vi "RX Detect Sync Error.vi"(0 "rx baseband session in":T2={"3630 session"={"VISA resource name"="", "Address Space"=1, "window_offset"=0, "register_addresses"={"MM based Registers"={"Revision"=0, "OldestCompatRev"=0, "signature"=0, "scratch"=0, "LedControl"=0, "BoardHwRev"=0, "BoardControl"=0, "ThermalStatus"=0, "BasebandStatus"=0, "BasebandControl"=0, "BasebandAuxSetup"=0, "BasebandAuxStatus"=0, "LmkSyncOutSetup"=0, " AdcSyncOutSetup"=0, " InjSyncOutSetup"=0, " PxiTrig0OutSetup"=0, " PxiTrig1OutSetup"=0, " PxiTrig2OutSetup"=0, " PxiTrig3OutSetup"=0, " PxiTrig4OutSetup"=0, " PxiTrig5OutSetup"=0, " PxiTrig6OutSetup"=0, " PxiTrig7OutSetup"=0}, "CPLD based Registers"={"SlaveSignature"=0, "SlaveRevision"=0, "SlaveOldestCompatRev"=0, "SlaveScratch"=0, "SlaveSetup"=0, "SlaveStatus"=0, "IDacReg_offset"=0, "LMKRegGrp0_offset"=0, "QDacReg_offset"=0, "BrdTempSensorVal"=0, "TempSensorPowerDown"=0, "GPIOReg_offset"=0, "IAdcReg_offset"=0, "QAdcReg_offset"=0, "LMKRegGrp1_offset"=0, "QadcTempSensorVal"=0, "IadcTempSensorVal"=0, "RevisionReg"=0, "VcxoReg"=0, "CpldStatusReg"=0, "PowerReg"=0, "VBiasEnReg"=0, "ExtRefOeReg"=0, "QdacCtrlReg"=0, "QdacStatusReg"=0, "IdacCtrlReg"=0, "IdacStatusReg"=0, "QdacJtagIn"=0, "QdacJtagOut"=0, "IdacJtagIn"=0, "IdacJtagOut"=0, "IqDcSetupReg"=0, "QadcStatusReg"=0, "IadcStatusReg"=0, "BrdSetupReg"=0, "IqDcRevisionReg"=0, "PllStatusReg"=0, "EndpointScratchReg"=0, "AdcSyncCfgReg"=0, "IqCardOpampReg"=0}, "CPLD Register Offset"=0, "MM  Register Offset"=0, " PxiTrig0OutSetup"=0}, "required_MM_fpga_version"={"signature"=0, "hardware"=0, "current revision"=0, "oldest revision"=0}, "CPLD Oldest Compat Version "={"hardware"=0, "CPLD firmware"=0}, "MM_FPGA_image_location"="", "is_init"=FALSE, "card_type"=enum."ADC", "DacLmkConfigFileName"="", "AdcLmkConfigFileName"="", "AdcConfigFileName"="", "DacConfigFileName_RevA"="", "DacConfigFileName_RevB"="", "Mulde hardware revision"=0, "bypass DAC PLL\n"=FALSE, "IQ Card Revision"=enum."RevA", "board capability"={"baseband sync"=enum."no baseband sync"}}, "7902 reference"=refnum} {"3630 session"."Address Space" items=["VXI/VME A16"=1, "VXI/VME A24"=2, "VXI/VME A32"=3, "VXI/VME A64"=4, "PXI Memory Allocations"=9, "PXI Configuration"=10, "PXI BAR0"=11, "PXI BAR1"=12, "PXI BAR2"=13, "PXI BAR3"=14, "PXI BAR4"=15, "PXI BAR5"=16]}, 5 "fpga reference in":refnum<k20>[](array[refnum]), 7 "direction":T1, 11 "error in":errorcluster) -> (4 "rx baseband session out":T2={"3630 session"={"VISA resource name"="", "Address Space"=1, "window_offset"=0, "register_addresses"={"MM based Registers"={"Revision"=0, "OldestCompatRev"=0, "signature"=0, "scratch"=0, "LedControl"=0, "BoardHwRev"=0, "BoardControl"=0, "ThermalStatus"=0, "BasebandStatus"=0, "BasebandControl"=0, "BasebandAuxSetup"=0, "BasebandAuxStatus"=0, "LmkSyncOutSetup"=0, " AdcSyncOutSetup"=0, " InjSyncOutSetup"=0, " PxiTrig0OutSetup"=0, " PxiTrig1OutSetup"=0, " PxiTrig2OutSetup"=0, " PxiTrig3OutSetup"=0, " PxiTrig4OutSetup"=0, " PxiTrig5OutSetup"=0, " PxiTrig6OutSetup"=0, " PxiTrig7OutSetup"=0}, "CPLD based Registers"={"SlaveSignature"=0, "SlaveRevision"=0, "SlaveOldestCompatRev"=0, "SlaveScratch"=0, "SlaveSetup"=0, "SlaveStatus"=0, "IDacReg_offset"=0, "LMKRegGrp0_offset"=0, "QDacReg_offset"=0, "BrdTempSensorVal"=0, "TempSensorPowerDown"=0, "GPIOReg_offset"=0, "IAdcReg_offset"=0, "QAdcReg_offset"=0, "LMKRegGrp1_offset"=0, "QadcTempSensorVal"=0, "IadcTempSensorVal"=0, "RevisionReg"=0, "VcxoReg"=0, "CpldStatusReg"=0, "PowerReg"=0, "VBiasEnReg"=0, "ExtRefOeReg"=0, "QdacCtrlReg"=0, "QdacStatusReg"=0, "IdacCtrlReg"=0, "IdacStatusReg"=0, "QdacJtagIn"=0, "QdacJtagOut"=0, "IdacJtagIn"=0, "IdacJtagOut"=0, "IqDcSetupReg"=0, "QadcStatusReg"=0, "IadcStatusReg"=0, "BrdSetupReg"=0, "IqDcRevisionReg"=0, "PllStatusReg"=0, "EndpointScratchReg"=0, "AdcSyncCfgReg"=0, "IqCardOpampReg"=0}, "CPLD Register Offset"=0, "MM  Register Offset"=0, " PxiTrig0OutSetup"=0}, "required_MM_fpga_version"={"signature"=0, "hardware"=0, "current revision"=0, "oldest revision"=0}, "CPLD Oldest Compat Version "={"hardware"=0, "CPLD firmware"=0}, "MM_FPGA_image_location"="", "is_init"=FALSE, "card_type"=enum."ADC", "DacLmkConfigFileName"="", "AdcLmkConfigFileName"="", "AdcConfigFileName"="", "DacConfigFileName_RevA"="", "DacConfigFileName_RevB"="", "Mulde hardware revision"=0, "bypass DAC PLL\n"=FALSE, "IQ Card Revision"=enum."RevA", "board capability"={"baseband sync"=enum."no baseband sync"}}, "7902 reference"=refnum} {"3630 session"."Address Space" items=["VXI/VME A16"=1, "VXI/VME A24"=2, "VXI/VME A32"=3, "VXI/VME A64"=4, "PXI Memory Allocations"=9, "PXI Configuration"=10, "PXI BAR0"=11, "PXI BAR1"=12, "PXI BAR2"=13, "PXI BAR3"=14, "PXI BAR4"=15, "PXI BAR5"=16]}, 8 "sync error":bool, 15 "error out":errorcluster)   [LabVIEW 2019]
uses:
  TypeDefs/Rx Baseband Session.ctl
  <instrlib>/niMmWave/ni3610 and ni3630/controls/public/Main Settings.ctl
  <vilib>/Instr/_visa.llb/VISA Register Access Address Space.ctl
  <instrlib>/niMmWave/ni3610 and ni3630/controls/public/Register Adresses.ctl
  <instrlib>/niMmWave/ni3610 and ni3630/controls/public/Base Card Type.ctl
  <instrlib>/niMmWave/ni3610 and ni3630/controls/private/IQ Card Revision.ctl
  <instrlib>/niMmWave/ni3610 and ni3630/controls/public/Board Capability.ctl
  TypeDefs/Blank FPGA Reference.ctl
  TypeDefs/Direction.ctl
  <vilib>/Analysis/5stat.llb/RMS (DBL).vi
  <vilib>/Analysis/baseanly.llb/Mean (CDB).vi
  <vilib>/Analysis/NI_AALPro.lvlib
  <vilib>/Analysis/NI_AALBase.lvlib
  <instrlib>/niMmWave/ni3610 and ni3630/ni3610_and_ni3630_Driver_Lib.lvlib
panel:
  out "data":dbl[][](graph)
  out "rms error":dbl[](array[numeric])
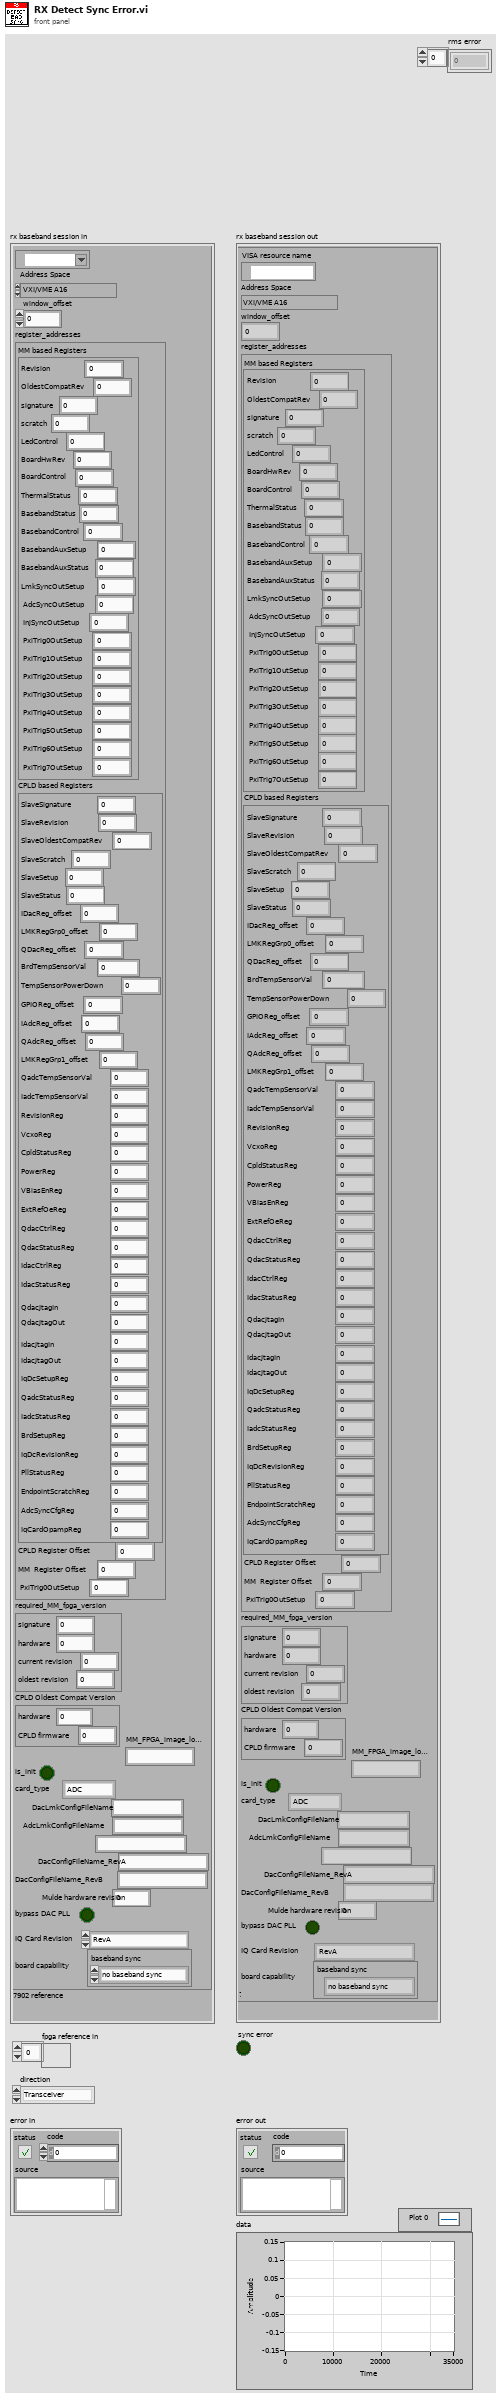
[diagram p1: front panel]
types:
  T1 = typedef "Direction.ctl" = enum16{"Transceiver", "Receiver", "Transmitter"}
  T2 = typedef "Rx Baseband Session.ctl" = cluster{"3630 session":T3, "7902 reference":T9}
  T3 = typedef "ni3610_and_ni3630_Driver_Lib.lvlib/Main Settings.ctl" = cluster{"VISA resource name":refnum<visa-resource-name>, "Address Space":T4, "window_offset":u32, "register_addresses":T5, "required_MM_fpga_version":cluster{"signature":u32, "hardware":u32, "current revision":u32, "oldest revision":u32}, "CPLD Oldest Compat Version ":cluster{"hardware":u32, "CPLD firmware":u32}, "MM_FPGA_image_location":string, "is_init":bool, "card_type":T6, "DacLmkConfigFileName":string, "AdcLmkConfigFileName":string, "AdcConfigFileName":string, "DacConfigFileName_RevA":string, "DacConfigFileName_RevB":string, "Mulde hardware revision":u8, "bypass DAC PLL\n":bool, "IQ Card Revision":T7, "board capability":T8}
  T4 = typedef "VISA Register Access Address Space.ctl" = u16
  T5 = typedef "ni3610_and_ni3630_Driver_Lib.lvlib/Register Adresses.ctl" = cluster{"MM based Registers":cluster{"Revision":u32, "OldestCompatRev":u32, "signature":u32, "scratch":u32, "LedControl":u32, "BoardHwRev":u32, "BoardControl":u32, "ThermalStatus":u32, "BasebandStatus":u32, "BasebandControl":u32, "BasebandAuxSetup":u32, "BasebandAuxStatus":u32, "LmkSyncOutSetup":u32, " AdcSyncOutSetup":u32, " InjSyncOutSetup":u32, " PxiTrig0OutSetup":u32, " PxiTrig1OutSetup":u32, " PxiTrig2OutSetup":u32, " PxiTrig3OutSetup":u32, " PxiTrig4OutSetup":u32, " PxiTrig5OutSetup":u32, " PxiTrig6OutSetup":u32, " PxiTrig7OutSetup":u32}, "CPLD based Registers":cluster{"SlaveSignature":u32, "SlaveRevision":u32, "SlaveOldestCompatRev":u32, "SlaveScratch":u32, "SlaveSetup":u32, "SlaveStatus":u32, "IDacReg_offset":u32, "LMKRegGrp0_offset":u32, "QDacReg_offset":u32, "BrdTempSensorVal":u32, "TempSensorPowerDown":u32, "GPIOReg_offset":u32, "IAdcReg_offset":u32, "QAdcReg_offset":u32, "LMKRegGrp1_offset":u32, "QadcTempSensorVal":u32, "IadcTempSensorVal":u32, "RevisionReg":u32, "VcxoReg":u32, "CpldStatusReg":u32, "PowerReg":u32, "VBiasEnReg":u32, "ExtRefOeReg":u32, "QdacCtrlReg":u32, "QdacStatusReg":u32, "IdacCtrlReg":u32, "IdacStatusReg":u32, "QdacJtagIn":u32, "QdacJtagOut":u32, "IdacJtagIn":u32, "IdacJtagOut":u32, "IqDcSetupReg":u32, "QadcStatusReg":u32, "IadcStatusReg":u32, "BrdSetupReg":u32, "IqDcRevisionReg":u32, "PllStatusReg":u32, "EndpointScratchReg":u32, "AdcSyncCfgReg":u32, "IqCardOpampReg":u32}, "CPLD Register Offset":u32, "MM  Register Offset":u32, " PxiTrig0OutSetup":u32}
  T6 = typedef "ni3610_and_ni3630_Driver_Lib.lvlib/Base Card Type.ctl" = enum16{"unspecified", "ADC", "DAC"}
  T7 = typedef "ni3610_and_ni3630_Driver_Lib.lvlib/IQ Card Revision.ctl" = enum16{"RevA", "RevB", "RevC", "RevD"}
  T8 = typedef "ni3610_and_ni3630_Driver_Lib.lvlib/Board Capability.ctl" = cluster{"baseband sync":enum16{"no baseband sync", "baseband sync"}}
  T9 = typedef "Blank FPGA Reference.ctl" = refnum<k20>
  T10 = enum16{"software", "external", "rising zero", "falling zero"}
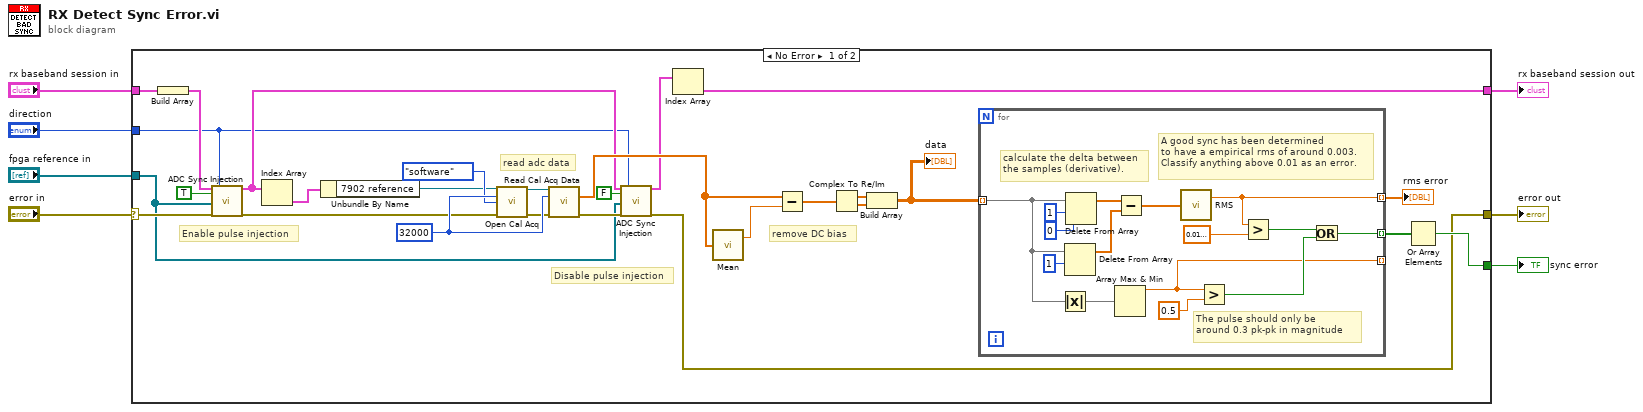
[diagram p0: block diagram]
diagram:
  n1 = case shown="No Error" "error in" {
    selector: "error in" -> [w18 w52]
    tunnel: [w16 w52] -> w7
    tunnel: [w31 _] -> w6
    tunnel: "rx baseband session in" -> [w15 w51]
    tunnel: [w10 w51] -> w3
    tunnel: "fpga reference in" -> [w9 _]
    tunnel: "direction" -> [w8 _]
    frame No Error {
      w29 = u16 32000 ("number of samples")
      # "remove DC bias"
      # "Disable pulse injection"
      # "read adc data"
      # "Enable pulse injection"
      n2 = Build Array(w15) -> (w14:T2[])
      n3 = call "ADC Sync Injection.vi"("rx baseband session in"=w14, "enable"=TRUE ("pxi trig 6 output enable"), "fpga reference in"=w9, "error in"=w18, "direction"=w8) -> ("rx baseband session out"=w12:T2[], "error out"=w24:errorcluster)  [unwired: 13 in]
      n4 = Index Array(array=w12) -> (element=w13:T2)  [unwired: 1 in]
      n5 = Unbundle By Name(w13) -> ("7902 reference"=w17:T9)
      n6 = call "Open Cal Acq.vi"("fpga reference in"=w17, "number of samples"=w29, "trigger type"=T10."software", "error in"=w24) -> ("fpga reference out"=w30:T9, "error out"=w28:errorcluster)  [unwired: 10 in]
      n7 = call "Read Cal Acq Data.vi"("fpga reference in"=w30, "number of samples"=w29, "error in"=w28) -> ("data"=w21:cdb[], "error out"=w22:errorcluster)  [unwired: 10 in, 1 out]
      n8 = call "ADC Sync Injection.vi"("rx baseband session in"=w12, "enable"=FALSE, "fpga reference in"=w9, "error in"=w22, "direction"=w8) -> ("rx baseband session out"=w11:T2[], "error out"=w16:errorcluster)  [unwired: 13 in]
      n9 = Index Array(array=w11) -> (element=w10:T2)  [unwired: 1 in]
      n10 = call-poly <vilib>:"Mean.vi"("X"=w21) -> ("mean"=w35:cdb)  [unwired: 1 out]
      n11 = Subtract(x=w21, y=w35) -> (x-y=w26:cdb[])
      n12 = Complex To Re/Im(x + iy=w26) -> (x=w34:dbl[], y=w33:dbl[])
      n13 = Build Array(w34, w33) -> (w19:dbl[][])
      "data" <- w19
      n14 = for {
        tunnel: w19 -> [w44] mode=indexing
        tunnel: [w42] -> w32 mode=indexing
        tunnel: [w39] -> w25 mode=indexing
        tunnel: [w36] -> _ mode=indexing
        # "The pulse should only be \naround 0.3 pk-pk in magnitude"
        # "A good sync has been determined\nto have a empirical rms of around 0.003.\nClassify anything above 0.01 as an error."
        # "calculate the delta between\nthe samples (derivative)."
        n15 = Absolute Value(x=w44) -> (abs(x)=w38:dbl[])
        n16 = Delete From Array(array=w44, length=1) -> (array with subset deleted=w46:dbl[])  [unwired: 1 in, 1 out]
        n17 = Delete From Array(array=w44, length=1, index=0) -> (array with subset deleted=w47:dbl[])  [unwired: 1 out]
        n18 = Array Max & Min(array=w38) -> (max value=w36:dbl)  [unwired: 3 out]
        n19 = Subtract(x=w47, y=w46) -> (x-y=w41:dbl[])
        n20 = call-poly <vilib>:"RMS.vi"("X"=w41) -> ("rms value"=w39:dbl)  [unwired: 1 out]
        n21 = Greater?(x=w36, y=0.5) -> (0:w37:bool)
        n22 = Greater?(x=w39, y=0.010000000000000002) -> (0:w40:bool)
        n23 = Or(x=w40, y=w37) -> (x .or. y?=w42:bool)
      }
      "rms error" <- w25
      n24 = Or Array Elements(Boolean array=w32) -> (logical OR=w31:bool)
    }
    frame Error {
    }
  }
  "error out" <- w7
  "sync error" <- w6
  "rx baseband session out" <- w3
